vi "UIMessage Callback.vi"(5 "Callback ID":i32, 7 "Owner":refnum<class>, 10 "User Data":variant, 11 "UIMessage":refnum<class "UIMessage.lvclass">) -> (0 "error out":errorcluster)   [LabVIEW 2020, in "TSnax.lvlib" / "Execution.lvclass"]
uses:
  Execution.lvclass
  UIMessage/UIMessage.lvclass
  Execution.lvclass/Execution.ctl
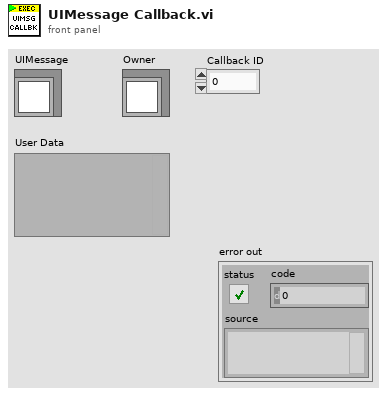
[diagram p1: front panel]
types:
  T1 = typedef "TSnax.lvlib/UIMsg.ctl" = enum16{"Unknown", "BreakOnUserRequest", "BreakOnBreakpoint", "BreakOnRunTimeError", "Trace", "TerminatingExecution", "AbortingExecution", "KillingExecutionThreads", "EndExecution", "ShutDownComplete", "StartExecution", "ProgressPercent", "ProgressText", "StartInteractiveExecution", "EndInteractiveExecution", "TerminatingInteractiveExecution", "TerminationCancelled", "ResumeFromBreak", "StartFileExecution", "EndFileExecution", "ShutDownCancelled", "LocalizationSettingChanged", "OpenWindows", "TileWindows", "CascadeWindows", "ReportChanged", "CloseWindows", "RefreshWindows", "ClientFileChanged", "DisplayReport", "ModelState_Initializing", "ModelState_Waiting", "ModelState_Identified", "ModelState_BeginTesting", "ModelState_TestingComplete", "ModelState_PostProcessingComplete", "ModelState_EnabledStateSet", "ReportLocationChanged", "GotoLocation", "PushUndoItem", "OutputMessages", "TypePaletteFileListChanged", "NonTerminatingThreadsArePreventingTermination", "ModelState_PostProcessing", "ReportCollectionChanged", "RuntimeError"}
  T2 = typedef "TSnax.lvlib/Execution.lvclass/Ref Data.ctl" = cluster{"Parameters":refnum<class "PropertyObject.lvclass">, "Client Sequence":refnum<class "SequenceFile.lvclass">, "Process Model":refnum<class "SequenceFile.lvclass">, "Entry Sequence":string, "Execution":refnum<k7>, "Report":refnum<class "Report.lvclass">, "Options":T3, "Started":bool, "Complete":bool}
  T3 = typedef "TSnax.lvlib/Execution Options.ctl" = cluster{"Use Default Model (T)":bool, "Release Related References (T)":bool}
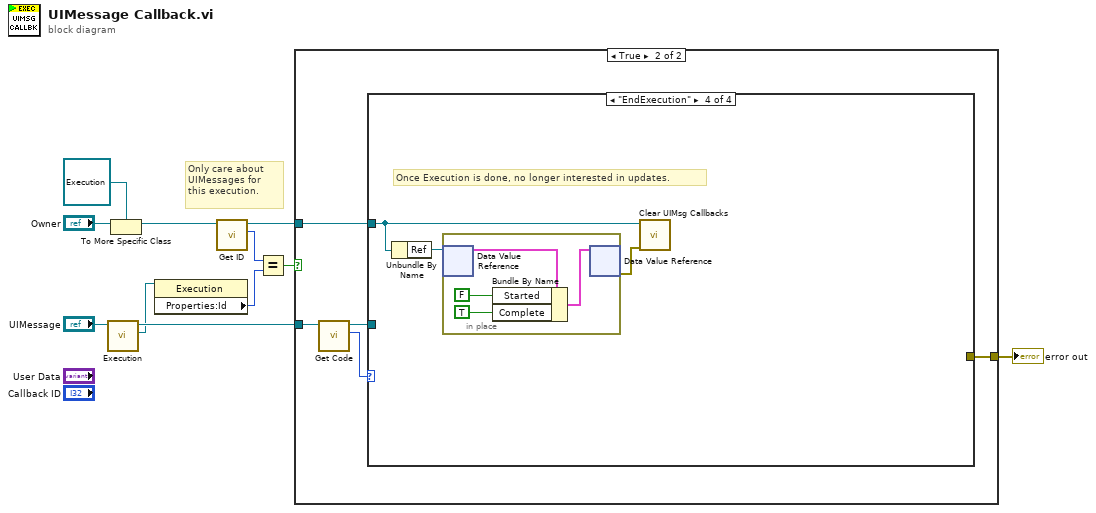
[diagram p0: block diagram]
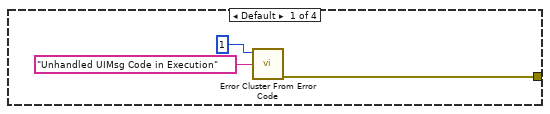
[diagram p3: hidden frame]
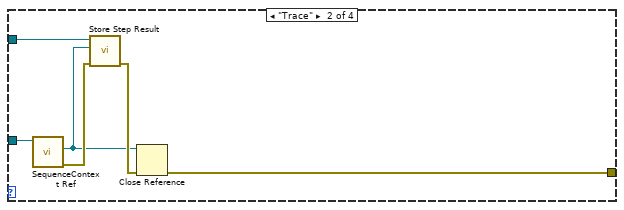
[diagram p4: hidden frame]
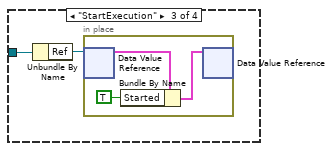
[diagram p5: hidden frame]
diagram:
  # "Only care about UIMessages for this execution."
  n1 = call "Execution.vi"("UIMessage in"="UIMessage") -> ("Execution"=w5:refnum<class "Execution.lvclass">, "UIMessage out"=w6:refnum<class "UIMessage.lvclass">)  [unwired: 8 in, 1 out]
  n2 = To More Specific Class(target class=refnum<class "Execution.lvclass"> refnum ("TSnax:Execution"), reference="Owner") -> (specific class reference=w3:refnum<class "Execution.lvclass">)  [unwired: 1 in, 1 out]
  n3 = property class="Execution"(reference=w5) -> ("Properties:Id"=w9:i32)  [unwired: 1 in, 2 out]
  n4 = call "Get ID.vi"("Execution in"=w3) -> ("Id"=w1:i32, "Execution out"=w2:refnum<class "Execution.lvclass">)  [unwired: 8 in, 1 out]
  n5 = Equal?(x=w1, y=w9) -> (x = y?=w8:bool)
  n6 = case shown="True" w8 {
    tunnel: w6 -> [_ w15]
    tunnel: w2 -> [_ w14]
    tunnel: [_ w12] -> w4
    frame False {
    }
    frame True {
      n7 = call "Get Code.vi"("UIMessage in"=w15) -> ("Code"=w16:T1, "UIMessage out"=w13:refnum<class "UIMessage.lvclass">)  [unwired: 8 in, 1 out]
      n8 = case shown="\"EndExecution\"" w16 {
        tunnel: w14 -> [_ w23 w26 w32]
        tunnel: w13 -> [_ w24 _ _]
        tunnel: [w17 w20 _ _] -> w12
        frame Default {
          n9 = call <vilib>:"Error Cluster From Error Code.vi"("error message (\"\")"="Unhandled UIMsg Code in Execution" ("error message (\"\")"), "error code (0)"=1) -> ("error out"=w17:errorcluster)  [unwired: 7 in]
        }
        frame "Trace" {
          n10 = call "SequenceContext Ref.vi"("UIMessage in"=w24) -> ("error out"=w22:errorcluster, "SequenceContext Ref"=w21:refnum<k7>)  [unwired: 8 in, 1 out]
          n11 = call "Store Step Result.vi"("error in (no error)"=w22, "SequenceContext Ref"=w21, "Execution in"=w23) -> ("error out"=w25:errorcluster)  [unwired: 7 in, 1 out]
          n12 = Close Reference(reference=w21, error in (no error)=w25) -> (error out=w20:errorcluster)
        }
        frame "StartExecution" {
          n13 = Unbundle By Name(w26) -> ("Ref"=w27:refnum<data-value>)
          n14 = in-place {
            n15 = in-place-dvr #1(w27) -> (w30:T2)  [unwired: 1 out]
            n16 = Bundle By Name(cluster=w30, "Started"=TRUE) -> (w29:T2)
            n17 = in-place-dvr #1(w29) -> ()  [unwired: 2 out]
          }
        }
        frame "EndExecution" {
          # "Once Execution is done, no longer interested in updates."
          n18 = Unbundle By Name(w32) -> ("Ref"=w33:refnum<data-value>)
          n19 = in-place {
            n20 = in-place-dvr #2(w33) -> (w37:T2)  [unwired: 1 out]
            n21 = Bundle By Name(cluster=w37, "Started"=FALSE, "Complete"=TRUE) -> (w36:T2)
            n22 = in-place-dvr #2(w36) -> (w31:errorcluster)  [unwired: 1 out]
          }
          n23 = call "Clear UIMsg Callbacks.vi"("error in (no error)"=w31, "Execution in"=w32) -> ()  [unwired: 8 in, 2 out]
        }
      }
    }
  }
  "error out" <- w4
